vi "1.3服务端创建.vi"() -> ()   [LabVIEW 2018]
panel:
  in  "数据输入":string
  out "数据输出":string
  in  "写":bool
  in  "读":bool
  in  "停止":bool
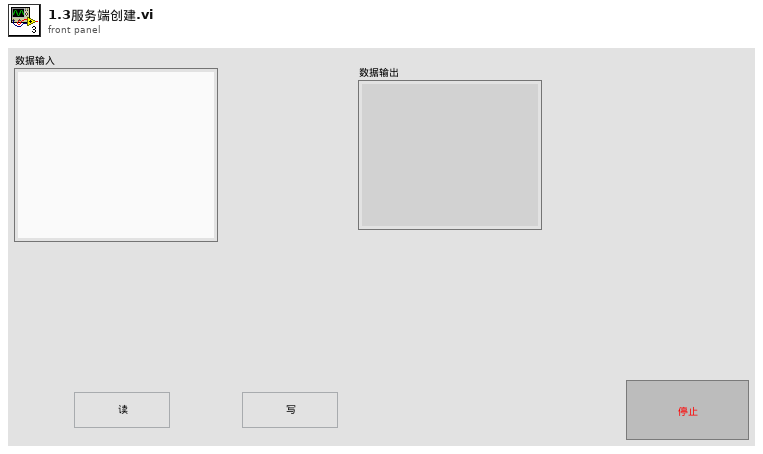
[diagram p1: front panel]
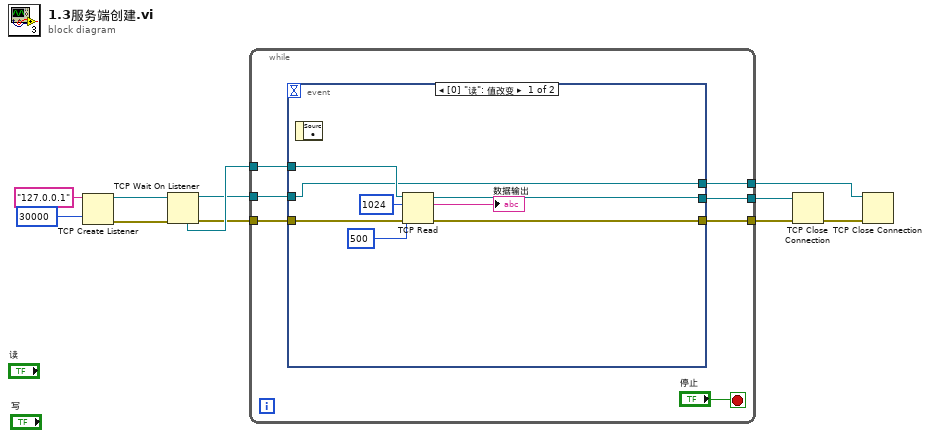
[diagram p0: block diagram]
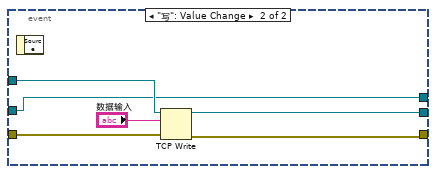
[diagram p2: hidden frame]
diagram:
  n1 = TCP Create Listener(10:u16 30000 ("端口"), 11:"127.0.0.1" ("服务名称")) -> (0:w8:errorcluster, 3:w9:refnum<k5>)  [unwired: 3 in, 1 out]
  n2 = TCP Wait On Listener(8:w8, 11:w9) -> (0:w6:errorcluster, 3:w5:refnum<k5>, 4:w7:refnum<k5>)  [unwired: 2 in, 2 out]
  n3 = while {
    tunnel: w7 -> [w17]
    tunnel: w6 -> [w16]
    tunnel: [w15] -> w4
    tunnel: w5 -> [w14]
    tunnel: [w13] -> w3
    tunnel: [w12] -> w2
    stop <- "停止" stop-if-true
    n4 = event shown="[0] \"读\": 值改变" {
      selector: _ -> [_ _]
      dyn-events: _ -> [_ _]
      timeout: _ -> [_ _]
      tunnel: w17 -> [w26 w30]
      tunnel: w16 -> [w25 w32]
      tunnel: [w24 w31] -> w15
      tunnel: w14 -> [w20 w27]
      tunnel: [w21 w28] -> w13
      tunnel: [w20 w27] -> w12
      event "读": Value Change {
        n5 = event-data() -> ()  [unwired: 1 in, 1 out]
        n6 = TCP Read(connection ID=w26, bytes to read=1024 ("读取的字节"), error in (no error)=w25, 9:500 ("超时毫秒(25000)")) -> (connection ID out=w21:refnum<k5>, data out=→"数据输出":string, error out=w24:errorcluster)  [unwired: 1 in]
      }
      event "写": Value Change {
        n7 = event-data() -> ()  [unwired: 1 in, 1 out]
        n8 = TCP Write(connection ID=w30, data in="数据输入", error in (no error)=w32) -> (connection ID out=w28:refnum<k5>, error out=w31:errorcluster)  [unwired: 1 in, 1 out]
      }
    }
  }
  n9 = TCP Close Connection(connection ID=w3, error in (no error)=w4) -> (error out=w1:errorcluster)  [unwired: 1 in, 1 out]
  n10 = TCP Close Connection(connection ID=w2, error in (no error)=w1) -> ()  [unwired: 1 in, 2 out]
